vi "EnumCases.vi"() -> ()   [LabVIEW 2019]
panel:
  in  "Week":T1(ring)
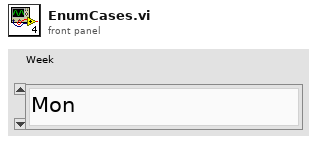
[diagram p1: front panel]
types:
  T1 = enum16{"Mon", "Tue", "Wed", "Thu", "Fir", "Sat", "Sun"}
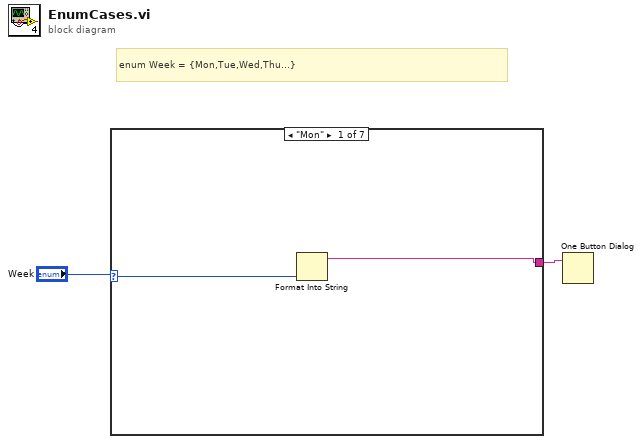
[diagram p0: block diagram]
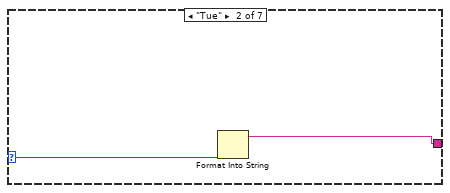
[diagram p2: hidden frame]
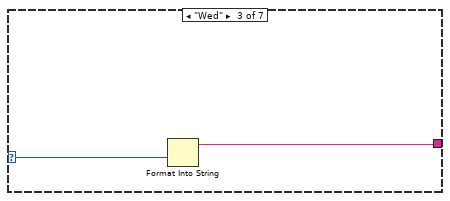
[diagram p3: hidden frame]
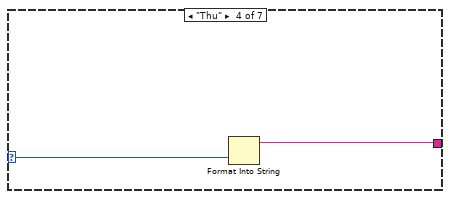
[diagram p4: hidden frame]
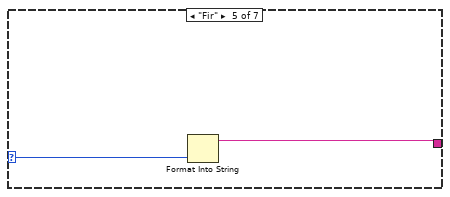
[diagram p5: hidden frame]
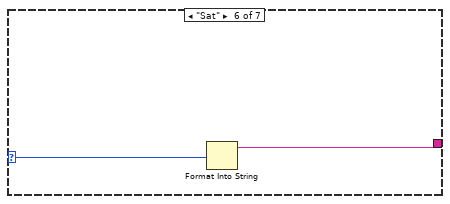
[diagram p6: hidden frame]
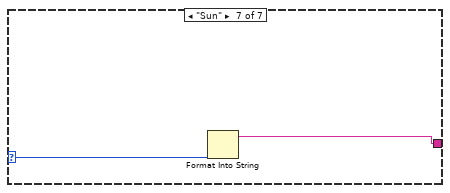
[diagram p7: hidden frame]
diagram:
  # "enum Week = {Mon,Tue,Wed,Thu...}"
  n1 = case shown="\"Mon\"" "Week" {
    selector: "Week" -> [w4 w6 w8 w10 w12 w14 w16]
    tunnel: [w3 w5 w7 w9 w11 w13 w15] -> w1
    frame "Mon" {
      n2 = Format Into String(w4) -> (resulting string=w3:string)  [unwired: 3 in, 1 out]
    }
    frame "Tue" {
      n3 = Format Into String(w6) -> (resulting string=w5:string)  [unwired: 3 in, 1 out]
    }
    frame "Wed" {
      n4 = Format Into String(w8) -> (resulting string=w7:string)  [unwired: 3 in, 1 out]
    }
    frame "Thu" {
      n5 = Format Into String(w10) -> (resulting string=w9:string)  [unwired: 3 in, 1 out]
    }
    frame "Fir" {
      n6 = Format Into String(w12) -> (resulting string=w11:string)  [unwired: 3 in, 1 out]
    }
    frame "Sat" {
      n7 = Format Into String(w14) -> (resulting string=w13:string)  [unwired: 3 in, 1 out]
    }
    frame "Sun" {
      n8 = Format Into String(w16) -> (resulting string=w15:string)  [unwired: 3 in, 1 out]
    }
  }
  n9 = One Button Dialog(message=w1) -> ()  [unwired: 1 in, 1 out]
